vi "TEB Get Message.vi"() -> (0 "Text":string, 1 "TEB Message Type":T1(ring)=enum."StopEvent=")   [LabVIEW 2010]
panel:
  in  "Timeout ms (-1)":i32=-1
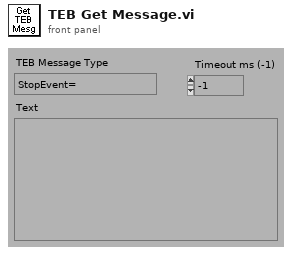
[diagram p1: front panel]
types:
  T1 = enum16{"No Message", "Bad Message", "Init", "StartEvent=", "EventFragment=", "InstantFragment=", "StopEvent=", "Processed=", "Address=", "Ping=", "Stop"}
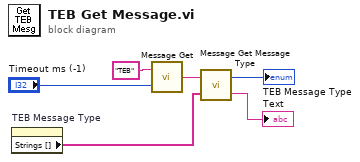
[diagram p0: block diagram]
diagram:
  n1 = property on="TEB Message Type" class="Enum (strict)"() -> ("Strings []"=w3:string[])  [unwired: 2 in, 2 out]
  n2 = call "Message Get.vi"("Timeout ms (-1)"="Timeout ms (-1)", "Module"="TEB") -> ("data out"=w4:string)
  n3 = call "Message Get Message Type.vi"("Message Types"=w3, "Message"=w4) -> ("Trailing text"=→"Text":string, "Message Type"=→"TEB Message Type":i32)
